vi "ZLIB Get File__ogtk.vi"(4 "password (none)":string, 5 "overwrite (F)":bool, 6 "error in (no error)":errorcluster, 7 "file info":T2 {"file timestamp" format="%<%H:%M:%S\n%d/%m/%Y>T"; "external fa" format="%.0x"; "internal fa" format="%.0x"; "crc" format="%.0x"}, 8 "target path":path, 9 "unzip Refnum":T1) -> (0 "error out":errorcluster, 3 "unzip Refnum out":T1)   [LabVIEW 2020]
doc: "Extracts the currently selected file inside the archive into an external file."
uses:
  <userlib>/_OpenG.lib/lvzip/lvzip.llb/ZLIB Unzip Handle__ogtk.ctl
  <userlib>/_OpenG.lib/lvzip/lvzip.llb/ZLIB File Info__ogtk.ctl
panel:
  # "Please visit http://www.OpenG.org to learn about the\nOpen Source LabVIEW software movement.\n\nNOTICE -- YOU MUST LEAVE THIS NOTICE IN PLACE.  PER THE TERMS OF THE LICENSE BELOW, YOU MAY SUBLICENSE THIS SOFTWARE \nIN ANY WAY THAT DOES NOT CONFLICT WITH THIS LICENSE.\n\n### BSD License (http://www.opensource.org/licenses/bsd-license.php) Begin ###\n \nCopyright (C) 2008 Rolf Kalbermatter rolf.kalbermatter@citeng.com\n\nAll rights reserved.\n\nRedistribution and use in source and binary forms, with or without modification, are permitted provided that the following conditions are met:\n\n    * Redistributions of source code must retain the above copyright notice, this list of conditions and the following disclaimer.\n    * Redistributions in binary form must reproduce the above copyright notice, this list of conditions and the following disclaimer in the \n       documentation and/or other materials provided with the distribution.\n    * Neither the name of SciWare, James Kring, Inc., nor the names of its contributors may be used to endorse or promote products derived \n       from this software without specific prior written permission.\n\nTHIS SOFTWARE IS PROVIDED BY THE COPYRIGHT HOLDERS AND CONTRIBUTORS \"AS IS\" AND ANY EXPRESS OR IMPLIED WARRANTIES, \nINCLUDING, BUT NOT LIMITED TO, THE IMPLIED WARRANTIES OF MERCHANTABILITY AND FITNESS FOR A PARTICULAR PURPOSE ARE \nDISCLAIMED. IN NO EVENT SHALL THE COPYRIGHT OWNER OR CONTRIBUTORS BE LIABLE FOR ANY DIRECT, INDIRECT, INCIDENTAL,\n SPECIAL, EXEMPLARY, OR CONSEQUENTIAL DAMAGES (INCLUDING, BUT NOT LIMITED TO, PROCUREMENT OF SUBSTITUTE GOODS OR \nSERVICES; LOSS OF USE, DATA, OR PROFITS; OR BUSINESS INTERRUPTION) HOWEVER CAUSED AND ON ANY THEORY OF LIABILITY, \nWHETHER IN CONTRACT, STRICT LIABILITY, OR TORT (INCLUDING NEGLIGENCE OR OTHERWISE) ARISING IN ANY WAY OUT OF THE USE \nOF THIS SOFTWARE, EVEN IF ADVISED OF THE POSSIBILITY OF SUCH DAMAGE.\n\n### BSD License End ###"
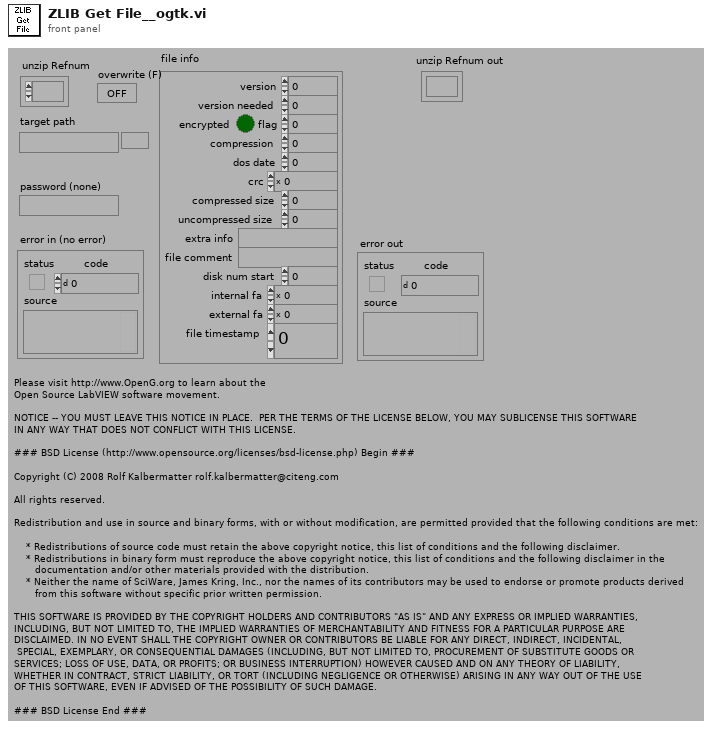
[diagram p1: front panel]
types:
  T1 = typedef "ZLIB Unzip Handle__ogtk.ctl" = refnum<k1>
  T2 = typedef "ZLIB File Info__ogtk.ctl" = cluster{"version":u32, "version needed":u32, "encrypted":bool, "flag":u32, "compression":i32, "dos date":u32, "crc":u32, "compressed size":u32, "uncompressed size":u32, "extra info":string, "file comment":string, "disk num start":u32, "internal fa":u32, "external fa":u32, "file timestamp":u32}
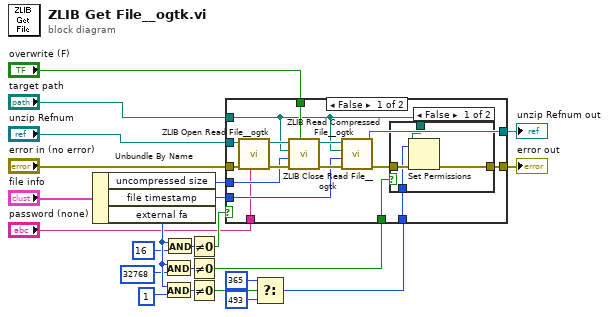
[diagram p0: block diagram]
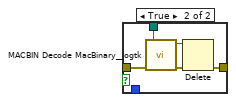
[diagram p2: hidden frame]
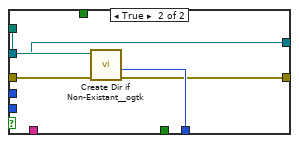
[diagram p3: hidden frame]
diagram:
  n1 = Unbundle By Name("file info") -> ("uncompressed size"=w3:u32, "file timestamp"=w15:u32, "external fa"=w21:u32)
  n2 = And(x=w21, y=u32 32768) -> (x .and. y?=w18:u32)
  n3 = And(x=w21, y=u32 1) -> (x .and. y?=w5:u32)
  n4 = And(x=w21, y=u32 16) -> (x .and. y?=w4:u32)
  n5 = Not Equal To 0?(x=w4) -> (x != 0?=w22:bool)
  n6 = Not Equal To 0?(x=w18) -> (x != 0?=w23:bool)
  n7 = Not Equal To 0?(x=w5) -> (x != 0?=w9:bool)
  n8 = Select(t=i16 365 ("new permissions"), s=w9, f=i16 493 ("new permissions")) -> (s? t:f=w10:i16)
  n9 = case shown="False" w22 {
    tunnel: "error in (no error)" -> [w38 w52]
    tunnel: w3 -> [w36 _]
    tunnel: "unzip Refnum" -> [w34 w49]
    tunnel: [w27 w48] -> w11
    tunnel: "target path" -> [w25 w51]
    tunnel: [w31 w49] -> w7
    tunnel: w10 -> [w24 w50]
    tunnel: "overwrite (F)" -> [w30 _]
    tunnel: w15 -> [w29 _]
    tunnel: "password (none)" -> [w28 _]
    tunnel: w23 -> [w26 _]
    frame False {
      n10 = call <userlib>:"ZLIB Open Read File__ogtk.vi"("password (none)"=w28, "error in (no error)"=w38, "unzip Refnum"=w34) -> ("error out"=w37:errorcluster, "unzip Refnum out"=w33:T1)  [unwired: 3 in, 2 out]
      n11 = call <userlib>:"ZLIB Read Compressed File__ogtk.vi"("overwrite (F)"=w30, "error in (no error)"=w37, "uncompressed size"=w36, "target path"=w25, "unzip Refnum"=w33) -> ("error out"=w35:errorcluster, "unzip Refnum out"=w32:T1)  [unwired: 3 in]
      n12 = call <userlib>:"ZLIB Close Read File__ogtk.vi"("error in (no error)"=w35, "file timestamp (no change)"=w29, "target path"=w25, "unzip Refnum"=w32) -> ("error out"=w27:errorcluster, "unzip Refnum out"=w31:T1)  [unwired: 6 in]
      n13 = case shown="False" w26 {
        tunnel: w27 -> [w41 w47]
        tunnel: [w40 w43] -> _
        tunnel: w25 -> [w42 w46]
        tunnel: w24 -> [w39 _]
        frame False {
          n14 = Set Permissions(7:w39, 8:w41, 11:w42) -> (0:w40:errorcluster)  [unwired: 2 in, 1 out]
        }
        frame True {
          n15 = call <userlib>:"MACBIN Decode MacBinary__ogtk.vi"("error in (no error)"=w47, "macbinary file"=w46) -> ("error out"=w44:errorcluster, "macbinary file out"=w45:path)  [unwired: 2 in, 2 out]
          n16 = Delete(path (use dialog)=w45, error in=w44) -> (error out=w43:errorcluster)  [unwired: 3 in, 2 out]
        }
      }
    }
    frame True {
      n17 = call <userlib>:"Create Dir if Non-Existant__ogtk.vi"("error in (no error)"=w52, "permissions (0755)"=w50, "Directory Path"=w51) -> ("error out"=w48:errorcluster)  [unwired: 6 in, 2 out]
    }
  }
  "error out" <- w11
  "unzip Refnum out" <- w7
